vi "Read Path.vi"(8 "error in (no error)":errorcluster, 11 "File IO.lvclass in":refnum<class "File IO.lvclass">) -> (0 "error out":errorcluster, 1 "File Path":path, 2 "Temporary Path":path, 3 "File IO.lvclass out":refnum<class "File IO.lvclass">, 4 "Settings Path":path)   [LabVIEW 2012, in "File IO.lvclass"]
uses:
  File IO.lvclass
  File IO.lvclass/File IO.ctl
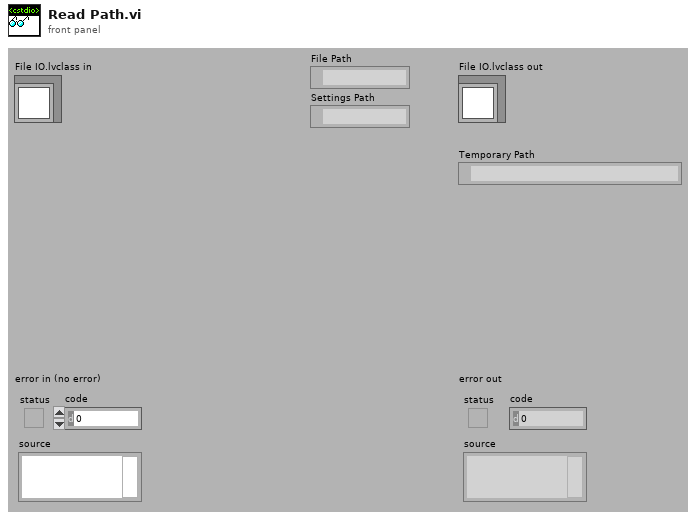
[diagram p1: front panel]
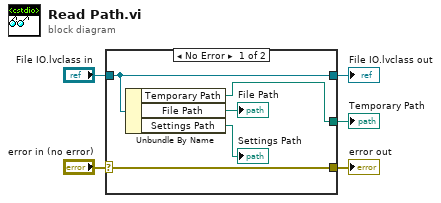
[diagram p0: block diagram]
diagram:
  n1 = case shown="No Error" "error in (no error)" {
    selector: "error in (no error)" -> [w10 w11]
    tunnel: [w10 w11] -> w4
    tunnel: [w9 w12] -> w2
    tunnel: "File IO.lvclass in" -> [w9 w12]
    tunnel: [w8 _] -> w1
    frame No Error {
      n2 = Unbundle By Name(w9) -> ("Temporary Path"=w8:path, "File Path"=→"File Path":path, "Settings Path"=→"Settings Path":path)
    }
    frame Error {
    }
  }
  "error out" <- w4
  "File IO.lvclass out" <- w2
  "Temporary Path" <- w1
